vi "Init.vi"(6 "Name (Caller VI)":string, 8 "error in (no error)":errorcluster) -> (0 "error out":errorcluster, 3 "2DArrayManager out":refnum<class "2DArrayManager.lvclass">)   [LabVIEW 2020, in "OOPanel.lvlib" / "2DArrayManager.lvclass"]
uses:
  2DArrayManager.lvclass
  Manager/Manager.lvclass
  ArrayPanel/ArrayPanel.lvclass
  2D Position.ctl
  OOPanel.lvlib
  2D Index.ctl
  Events.ctl
  Event Reg Ref.ctl
  Options.ctl
  State.ctl
  Direction.ctl
  Synced Scroll.ctl
  Update Data.ctl
  2DPanelBlank/2DPanelBlank.lvclass
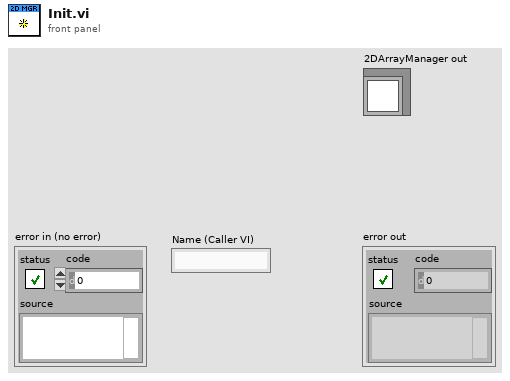
[diagram p1: front panel]
types:
  T1 = typedef "OOPanel.lvlib/2DArrayManager.lvclass/Update Data.ctl" = cluster{"Synced":bool, "Sync Response":refnum<notifier>}
  T2 = typedef "OOPanel.lvlib/2DArrayManager.lvclass/Synced Scroll.ctl" = cluster{"Position":T3, "Direction":T4, "Sync Response":refnum<notifier>}
  T3 = typedef "OOPanel.lvlib/2D Position.ctl" = cluster{"H":i32, "V":i32}
  T4 = typedef "OOPanel.lvlib/Direction.ctl" = enum16{"Vertical", "Horizontal", "Both"}
  T5 = typedef "OOPanel.lvlib/2DArrayManager.lvclass/State.ctl" = cluster{"Scroll":T3, "Scroll Max":T3, "Top-Left Index":T6, "H Scroll Sync":refnum<user-event>, "V Scroll Sync":refnum<user-event>, "Sync":bool, "H Scroll Vis":bool, "V Scroll Vis":bool, "Blank Pool":refnum<queue>}
  T6 = typedef "OOPanel.lvlib/2D Index.ctl" = cluster{"Row":i32, "Col":i32}
  T7 = typedef "OOPanel.lvlib/2DArrayManager.lvclass/Events.ctl" = cluster{"Stop":refnum<user-event>, "Update":refnum<user-event>, "Set BG":refnum<user-event>, "Scroll":refnum<user-event>, "Highlight":refnum<user-event>, "Synced Scroll":refnum<user-event>, "Scrollbars":refnum<user-event>}
  T8 = typedef "OOPanel.lvlib/2DArrayManager.lvclass/Options.ctl" = cluster{"Running":bool, "Borders":bool, "Background":u32, "V Scroll":bool, "H Scroll":bool, "Blank":refnum<class "2DPanelBlank.lvclass">, "Initial Blank Count":i32}
  T9 = typedef "OOPanel.lvlib/2DArrayManager.lvclass/Event Reg Ref.ctl" = cluster{"Last Update Ticks ms":u32, "Event Reg":refnum<event-registration>}
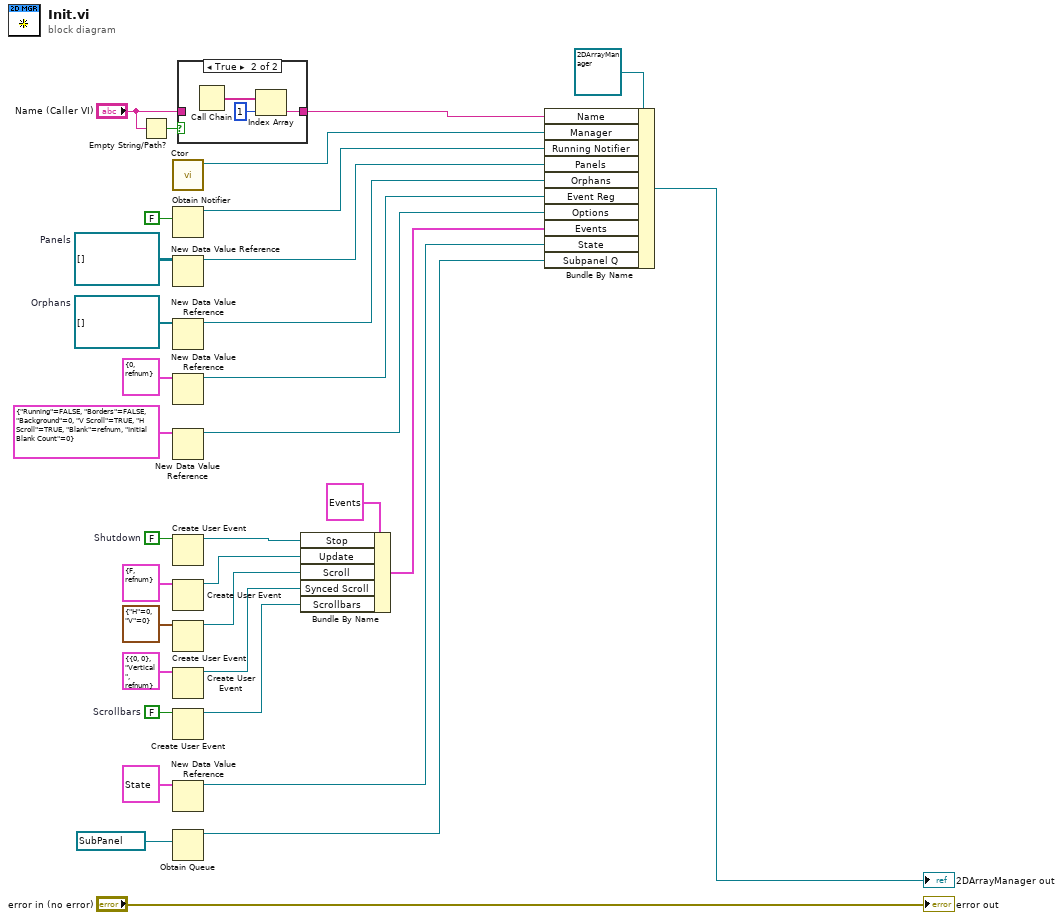
[diagram p0: block diagram]
diagram:
  w4 = FALSE  # Scrollbars
  w24 = refnum<class "ArrayPanel.lvclass">[] []  # Orphans
  w25 = refnum<class "ArrayPanel.lvclass">[][] []  # Panels
  w26 = FALSE  # Shutdown
  n1 = Empty String/Path?(string/path="Name (Caller VI)") -> (empty?=w30:bool)
  n2 = call "Ctor.vi"() -> ("Manager out"=w27:refnum<class "Manager.lvclass">)  [unwired: 10 in, 1 out]
  n3 = Obtain Notifier(notification data type=FALSE) -> (notifier out=w22:refnum<notifier>)  [unwired: 3 in, 2 out]
  n4 = New Data Value Reference(data value=w25) -> (data value reference=w21:refnum<data-value>)  [unwired: 1 in, 1 out]
  n5 = New Data Value Reference(data value=w24) -> (data value reference=w20:refnum<data-value>)  [unwired: 1 in, 1 out]
  n6 = New Data Value Reference(data value=T9 {"Last Update Ticks ms"=0, "Event Reg"=refnum} ("Event Reg Ref")) -> (data value reference=w18:refnum<data-value>)  [unwired: 1 in, 1 out]
  n7 = New Data Value Reference(data value=T8 {"Running"=FALSE, "Borders"=FALSE, "Background"=0, "V Scroll"=TRUE, "H Scroll"=TRUE, "Blank"=refnum, "Initial Blank Count"=0} ("State Ref")) -> (data value reference=w16:refnum<data-value>)  [unwired: 1 in, 1 out]
  n8 = Create User Event(user event datatype=w26) -> (user event=w13:refnum<user-event>)  [unwired: 1 in, 1 out]
  n9 = Create User Event(user event datatype=T1 {"Synced"=FALSE, "Sync Response"=refnum} ("Update Data")) -> (user event=w12:refnum<user-event>)  [unwired: 1 in, 1 out]
  n10 = Create User Event(user event datatype=T3 {"H"=0, "V"=0} ("Position")) -> (user event=w11:refnum<user-event>)  [unwired: 1 in, 1 out]
  n11 = Create User Event(user event datatype=T2 {"Position"={"H"=0, "V"=0}, "Direction"=enum."Vertical", "Sync Response"=refnum} ("Synced Scroll")) -> (user event=w6:refnum<user-event>)  [unwired: 1 in, 1 out]
  n12 = Create User Event(user event datatype=w4) -> (user event=w3:refnum<user-event>)  [unwired: 1 in, 1 out]
  n13 = New Data Value Reference(data value=T5 {"Scroll"={"H"=0, "V"=0}, "Scroll Max"={"H"=0, "V"=0}, "Top-Left Index"={"Row"=0, "Col"=0}, "H Scroll Sync"=refnum, "V Scroll Sync"=refnum, "Sync"=FALSE, "H Scroll Vis"=FALSE, "V Scroll Vis"=FALSE, "Blank Pool"=refnum} ("State")) -> (data value reference=w8:refnum<data-value>)  [unwired: 1 in, 1 out]
  n14 = Obtain Queue(element data type=refnum<vi> refnum ("target class")) -> (queue out=w1:refnum<queue>)  [unwired: 4 in, 2 out]
  n15 = case shown="True" w30 {
    tunnel: "Name (Caller VI)" -> [w34 _]
    tunnel: [w34 w35] -> w28
    frame False {
    }
    frame True {
      n16 = Call Chain() -> (call chain=w37:string[])
      n17 = Index Array(array=w37, index=1) -> (element=w35:string)
    }
  }
  n18 = Bundle By Name(cluster=T7 {"Stop"=refnum, "Update"=refnum, "Set BG"=refnum, "Scroll"=refnum, "Highlight"=refnum, "Synced Scroll"=refnum, "Scrollbars"=refnum} ("Events"), "Stop"=w13, "Update"=w12, "Scroll"=w11, "Synced Scroll"=w6, "Scrollbars"=w3) -> (w10:T7)
  n19 = Bundle By Name(cluster=refnum<class "2DArrayManager.lvclass"> refnum ("2DArrayManager in"), "Name"=w28, "Manager"=w27, "Running Notifier"=w22, "Panels"=w21, "Orphans"=w20, "Event Reg"=w18, "Options"=w16, "Events"=w10, "State"=w8, "Subpanel Q"=w1) -> (→"2DArrayManager out":refnum<class "2DArrayManager.lvclass">)
  "error out" <- "error in (no error)"
